vi "Replicate If.vi"(8 "If":T1[](array[typedef]), 9 "Replicate":T1[](array[typedef]), 10 "1D Maze":i32[](array[numeric]), 11 "Class":refnum<class "Pinwheel.lvclass">) -> (0 "Replicated":refnum<class "Pinwheel.lvclass">, 1 "Action":T2, 2 "Direction":T1, 3 "Class":refnum<class "Pinwheel.lvclass">)   [LabVIEW 2020, in "Pinwheel.lvclass"]
uses:
  Pinwheel.lvclass
  Type Defs/Direction Enum.ctl
  Type Defs/Action Enum.ctl
  Type Defs/SB Type Defs.lvlib
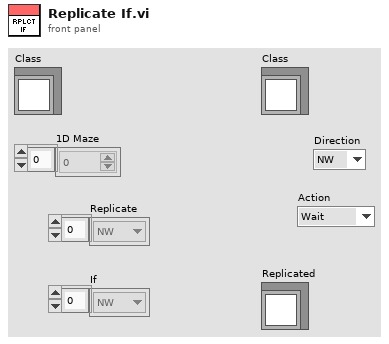
[diagram p1: front panel]
types:
  T1 = typedef "SB Type Defs.lvlib/Direction Enum.ctl" = enum16{"NW", "N", "NE", "E", "SE", "S", "SW", "W"}
  T2 = typedef "SB Type Defs.lvlib/Action Enum.ctl" = enum16{"Wait", "Move", "Attack", "Replicate"}
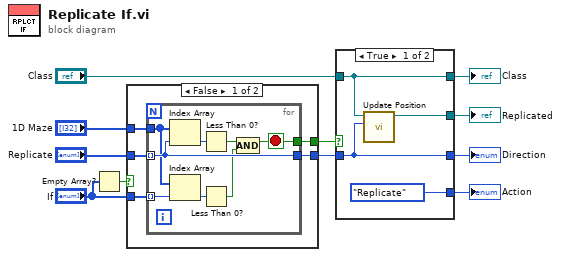
[diagram p0: block diagram]
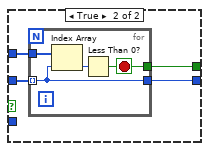
[diagram p2: hidden frame]
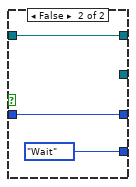
[diagram p3: hidden frame]
diagram:
  n1 = Empty Array?(array="If") -> (empty?=w2:bool)
  n2 = case shown="False" w2 {
    tunnel: "Replicate" -> [w16 w28]
    tunnel: [w15 w27] -> w5
    tunnel: [w14 w26] -> w6
    tunnel: "1D Maze" -> [w13 w25]
    tunnel: "If" -> [w12 _]
    frame False {
      n3 = for {
        tunnel: [w18] -> w14
        tunnel: w13 -> [w22]
        tunnel: [w23] -> w15
        tunnel: w16 -> [w23] mode=indexing
        tunnel: w12 -> [w21] mode=indexing
        stop <- w18 stop-if-true
        n4 = Index Array(array=w22, index=w23) -> (element=w24:i32)
        n5 = Index Array(array=w22, index=w21) -> (element=w20:i32)
        n6 = Less Than 0?(x=w24) -> (x < 0?=w19:bool)
        n7 = Less Than 0?(x=w20) -> (x < 0?=w17:bool)
        n8 = Compound Arithmetic op=AND(w19, w17) -> (w18:bool)
      }
    }
    frame True {
      n9 = for {
        tunnel: [w29] -> w26
        tunnel: w25 -> [w30]
        tunnel: [w31] -> w27
        tunnel: w28 -> [w31] mode=indexing
        stop <- w29 stop-if-true
        n10 = Index Array(array=w30, index=w31) -> (element=w32:i32)
        n11 = Less Than 0?(x=w32) -> (x < 0?=w29:bool)
      }
    }
  }
  n12 = case shown="True" w6 {
    tunnel: "Class" -> [w34 w37]
    tunnel: [Action_Enum."Replicate" ("Action") Action_Enum."Wait" ("Action")] -> w9
    tunnel: w5 -> [w35 w38]
    tunnel: [w35 w38] -> w10
    tunnel: [w34 w37] -> w11
    tunnel: [w33 _] -> w7
    frame True {
      n13 = call "Update Position.vi"("Direction"=w35, "Class"=w34) -> ("Class"=w33:refnum<class "Pinwheel.lvclass">)  [unwired: 9 in]
    }
    frame False {
    }
  }
  "Class" <- w11
  "Direction" <- w10
  "Action" <- w9
  "Replicated" <- w7
